vi "connect.vi"(8 "error in (no error)":errorcluster, 11 "RemoteAnalysisToolKit in":refnum<class "RemoteAnalysisToolKit.lvclass">) -> (0 "error out":errorcluster, 3 "RemoteAnalysisToolKit out":refnum<class "RemoteAnalysisToolKit.lvclass">)   [LabVIEW 2010, in "RemoteAnalysisToolKit.lvclass"]
uses:
  RemoteAnalysisToolKit.lvclass
  RemoteAnalysisToolKit.lvclass/RemoteAnalysisToolKit.ctl
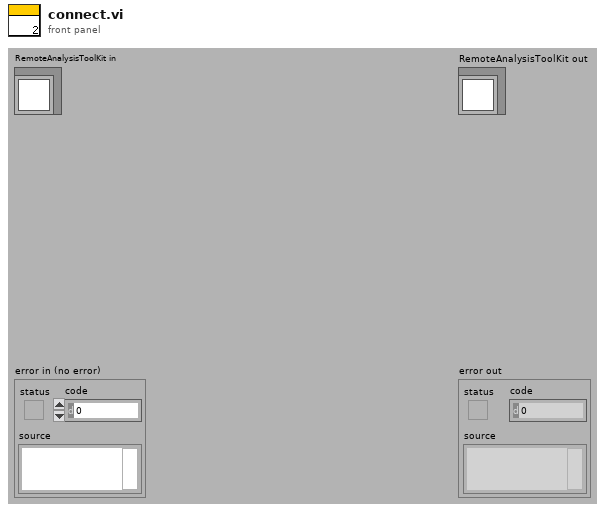
[diagram p1: front panel]
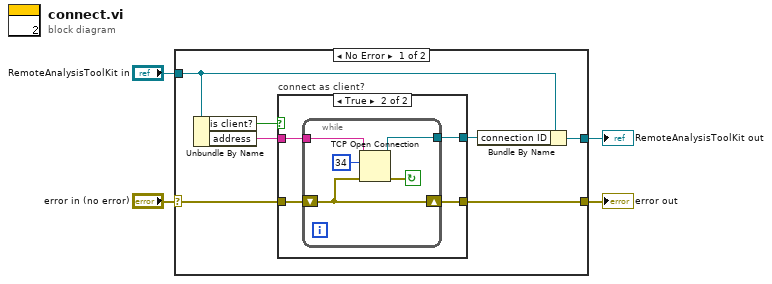
[diagram p0: block diagram]
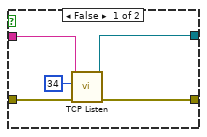
[diagram p2: hidden frame]
diagram:
  n1 = case shown="No Error" "error in (no error)" {
    selector: "error in (no error)" -> [w11 w27]
    tunnel: [w10 w27] -> w3
    tunnel: [w5 w26] -> w1
    tunnel: "RemoteAnalysisToolKit in" -> [w6 w26]
    frame No Error {
      n2 = Unbundle By Name(w6) -> ("is client?"=w9:bool, "address"=w8:string)
      n3 = case "connect as client?" shown="True" w9 {
        tunnel: w11 -> [w16 w20]
        tunnel: [w12 w19] -> w10
        tunnel: [w13 w18] -> w7
        tunnel: w8 -> [w15 w17]
        frame False {
          n4 = call <vilib>:"TCP Listen.vi"("error in (no error)"=w16, "port"=u16 34, "service name"=w15) -> ("error out"=w12:errorcluster, "connection ID"=w13:refnum<k5>)  [unwired: 5 in, 2 out]
        }
        frame True {
          n5 = while {
            tunnel: w17 -> [w24]
            tunnel: [w21] -> w18
            shift-right: [w22] -> w19
            shift-left: w20 -> [w22]
            stop <- w23 continue-if-true
            n6 = TCP Open Connection(address=w24, remote port or service name=u16 34, error in (no error)=w22) -> (connection ID=w21:refnum<k5>, error out=w23:errorcluster)  [unwired: 2 in]
          }
        }
      }
      n7 = Bundle By Name(cluster=w6, "connection ID"=w7) -> (w5:refnum<class "RemoteAnalysisToolKit.lvclass">)
    }
    frame Error {
    }
  }
  "error out" <- w3
  "RemoteAnalysisToolKit out" <- w1
